vi "K_S30_VISA Global.vi"() -> ()   [LabVIEW 2013, in "K_S30c_VISA.lvlib"]
uses:
  K_S30c_VISA.lvlib
panel:
  in  "RS-converter:\necho":bool=TRUE
  in  "VISA resource":refnum<visa-resource-name>="COM2"
  # "Global Variable for KELLER S30 driver Labview"
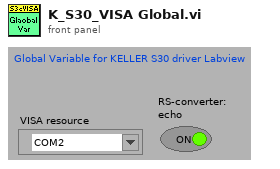
[diagram p1: front panel]
diagram:
